vi "setColorToDocument.vi"(8 "error in (no error)":errorcluster, 11 "xwpfRun in":refnum<class "xwpfRun.lvclass">) -> (0 "error out":errorcluster, 3 "xwpfRun out":refnum<class "xwpfRun.lvclass">)   [LabVIEW 2017, in "Word_Specific.lvlib" / "xwpfRun.lvclass"]
uses:
  xwpfRun.lvclass
  xwpfRun.lvclass/xwpfRun.ctl
  C:/Users/Neo/Desktop/Dev_Tools_BR/LabVIEW_NPOI/src/lib/NPOI 2.1.1/NPOI.OOXML.dll
  lib/NPOI 2.1.1/NPOI.OOXML.dll
  Styles/Style/Style.lvclass
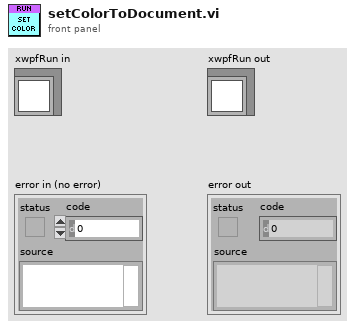
[diagram p1: front panel]
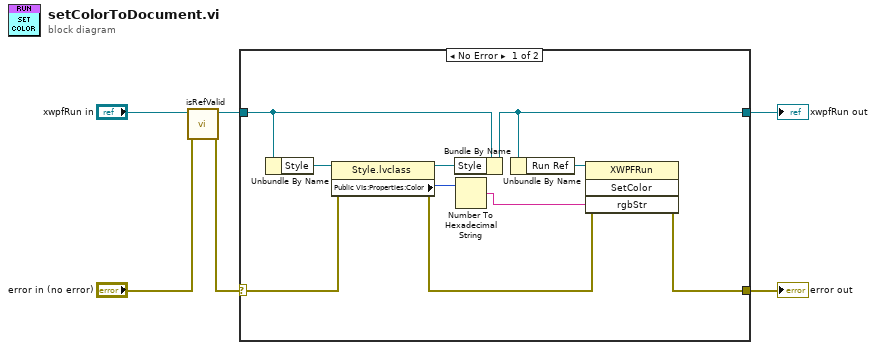
[diagram p0: block diagram]
diagram:
  n1 = call-dynamic "isRefValid.vi"("error in (no error)"="error in (no error)", "xwpfRun in"="xwpfRun in") -> ("error out"=w1:errorcluster, "xwpfRun out"=w3:refnum<class "xwpfRun.lvclass">)  [unwired: 8 in]
  n2 = case shown="No Error" w1 {
    selector: w1 -> [w12 w18]
    tunnel: [w7 w18] -> w6
    tunnel: [w11 w17] -> w4
    tunnel: w3 -> [w16 w17]
    frame No Error {
      n3 = Unbundle By Name(w16) -> ("Style"=w14:refnum<class "Style.lvclass">)
      n4 = property class="Style.lvclass"(reference=w14, error in=w12) -> (reference out=w13:refnum<class "Style.lvclass">, error out=w8:errorcluster, "Public VIs:Properties:Color"=w10:u32)
      n5 = Bundle By Name(cluster=w16, "Style"=w13) -> (w11:refnum<class "xwpfRun.lvclass">)
      n6 = Number To Hexadecimal String(2:w10) -> (0:w9:string)  [unwired: 1 in]
      n7 = Unbundle By Name(w11) -> ("Run Ref"=w15:refnum<k24>)
      n8 = invoke class="XWPFRun" method="SetColor"(reference=w15, error in=w8, "rgbStr"=w9) -> (error out=w7:errorcluster)  [unwired: 1 in, 3 out]
    }
    frame Error {
    }
  }
  "error out" <- w6
  "xwpfRun out" <- w4
